vi "Do TLS Upgrade.vi"(8 "error in (no error)":errorcluster, 10 "TCP In":refnum<k5>, 11 "Server in":refnum<class "Server.lvclass">) -> (0 "error out":errorcluster, 2 "TCP":refnum<k5>, 3 "Server out":refnum<class "Server.lvclass">)   [LabVIEW 2020, in "HTTP Server.lvlib" / "Server.lvclass"]
uses:
  Server.lvclass
  Server.lvclass/Server.ctl
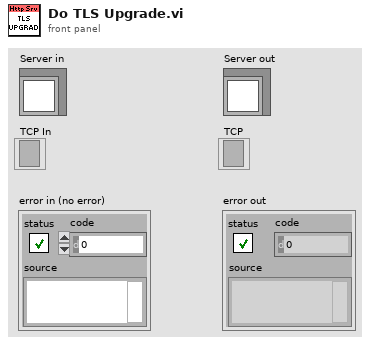
[diagram p1: front panel]
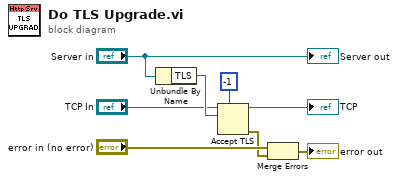
[diagram p0: block diagram]
diagram:
  n1 = Unbundle By Name("Server in") -> ("TLS"=w4:refnum<k36>)
  n2 = Accept TLS(7:-1 ("timeout ms"), 10:w4, 11:"TCP In") -> (0:w5:errorcluster, 3:→"TCP":refnum<k5>)  [unwired: 1 in, 1 out]
  n3 = Merge Errors("error in (no error)", w5) -> (→"error out":errorcluster)
  "Server out" <- "Server in"
